vi "principal.vi"() -> ()   [LabVIEW 2018]
uses:
  <vilib>/Instr/_visa.llb/Select Event Type.ctl
  <vilib>/Instr/_visa.llb/VISA Configure Serial Port (Instr).vi
  variables_globales.vi
panel:
  out "Waveform Chart 3":dbl(graph)
  out "Waveform Chart 2":dbl(graph)
  out "Waveform Chart":dbl(graph)
  in  "Seleccione el puerto serial":refnum<visa-resource-name>
  in  "stop":bool
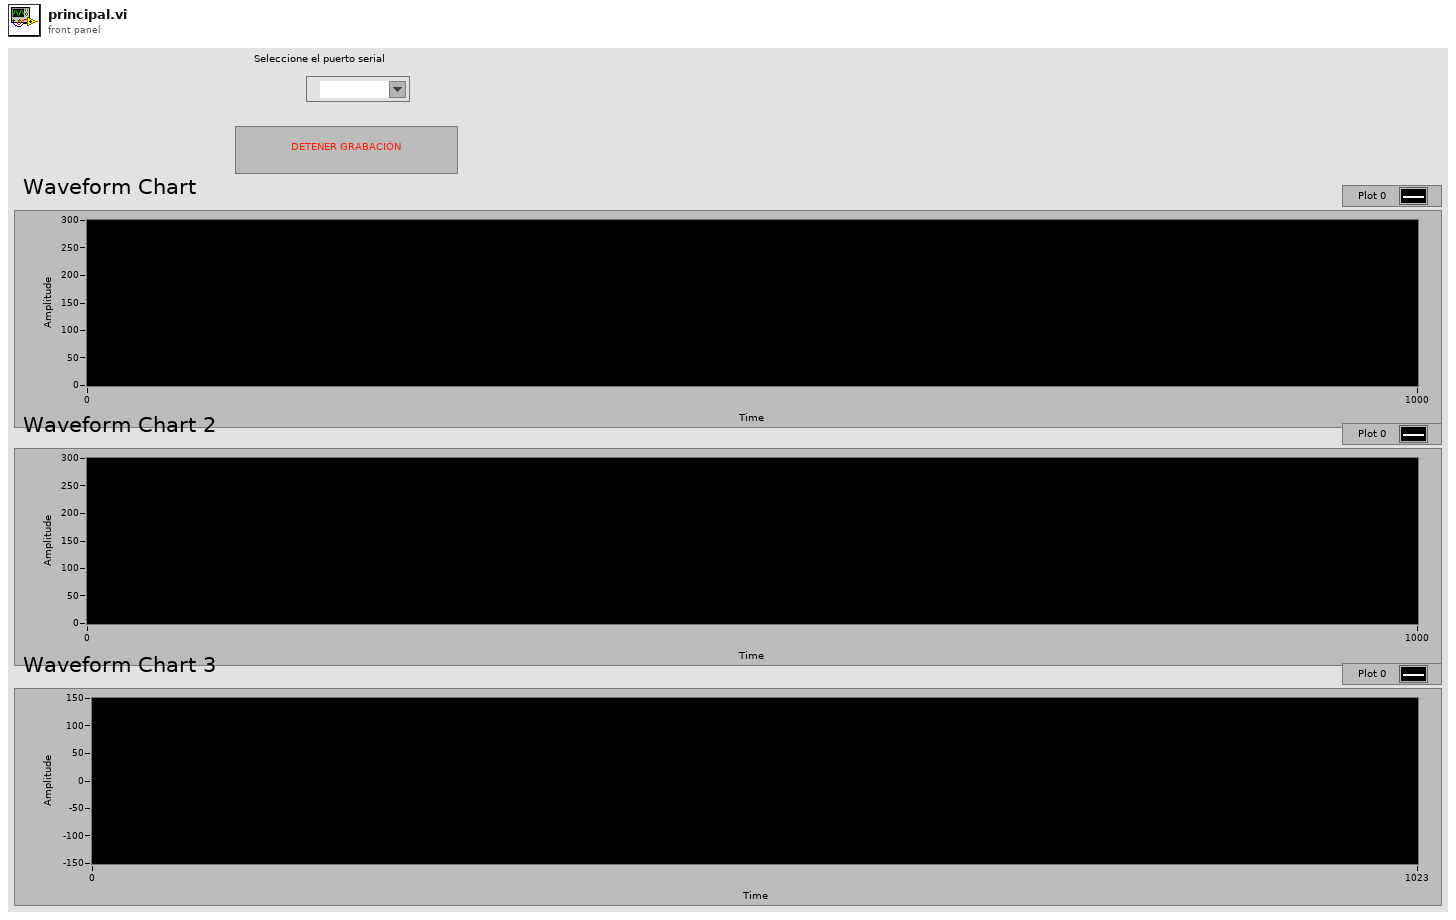
[diagram p1: front panel]
types:
  T1 = typedef "Select Event Type.ctl" = u32
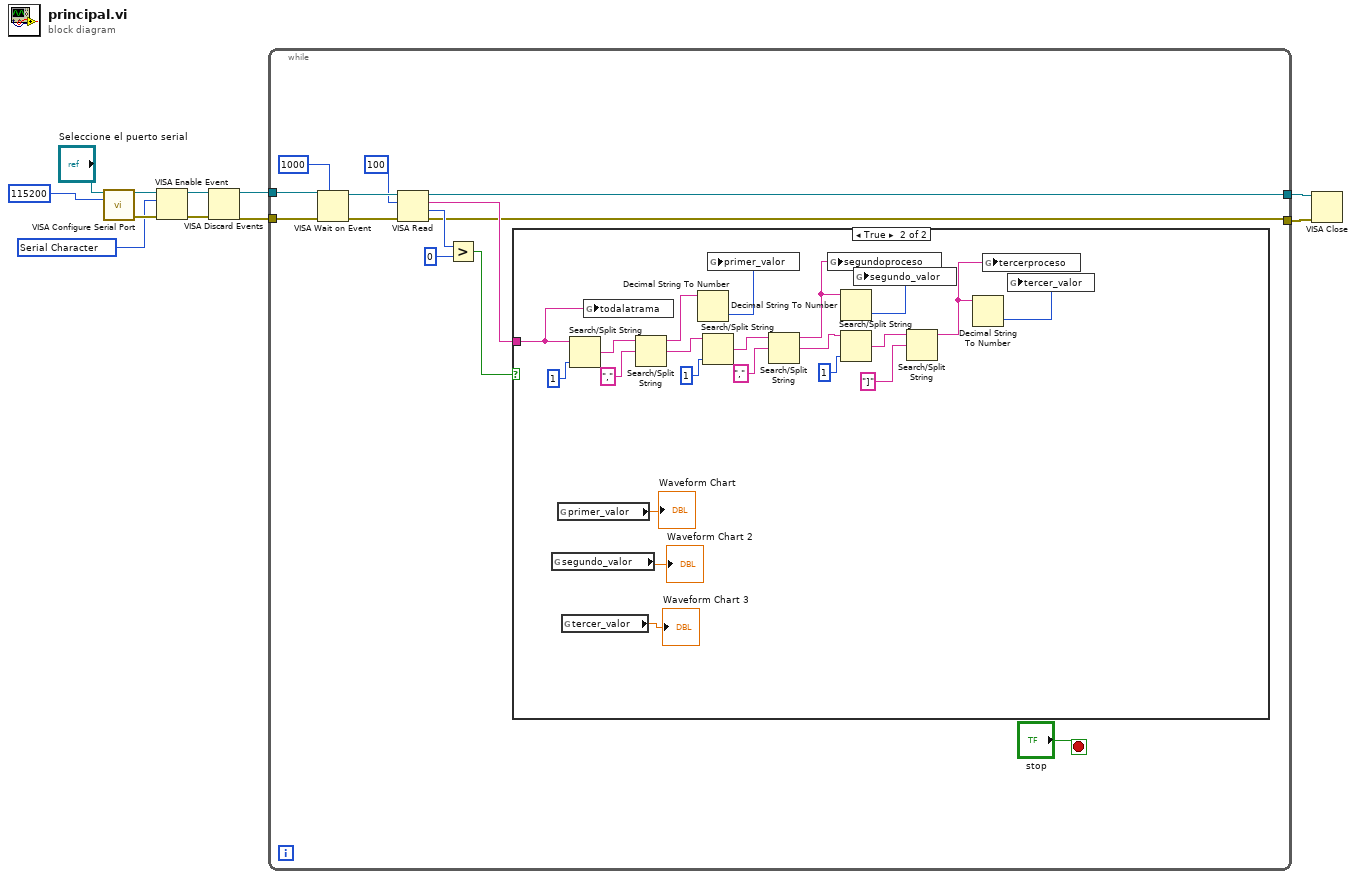
[diagram p0: block diagram]
diagram:
  w7 = T1 1073684533 items=["Service Request"=1073684491, "Trigger"=3221168138, "Clear"=1073684493, "VXI Signal"=1073684512, "VXI/VME Interrupt"=3221168161, "VXI/VME Sysfail"=1073684509, "VXI/VME Sysreset"=1073684510, "GPIB CIC"=1073684498, "GPIB Talk"=1073684499, "GPIB Listen"=1073684500, "PXI Interrupt"=1073684514, "Serial Break"=1073684515, "Serial TermChar"=1073684516, "Serial CTS"=1073684521, "Serial DSR"=1073684522, "Serial DCD"=1073684524, "Serial RI"=1073684526, "Serial Character"=1073684533, "USB Interrupt"=1073684535, "All Enabled"=1073709055] ("Event Type")
  n1 = call-poly "VISA Configure Serial Port"("VISA resource name"="Seleccione el puerto serial", "baud rate (9600)"=u32 115200) -> ("VISA resource name out"=w9:refnum<visa-resource-name>, "error out"=w8:errorcluster)  [unwired: 12 in]
  n2 = VISA Enable Event(8:w8, 10:w7, 11:w9) -> (0:w6:errorcluster, 3:w5:refnum<visa-resource-name>)  [unwired: 1 in]
  n3 = VISA Discard Events(8:w6, 11:w5) -> (0:w3:errorcluster, 3:w4:refnum<visa-resource-name>)  [unwired: 2 in]
  n4 = while {
    tunnel: w4 -> [w23]
    tunnel: w3 -> [w22]
    tunnel: [w13] -> w2
    tunnel: [w12] -> w1
    stop <- "stop" stop-if-true
    n5 = VISA Wait on Event(7:u32 1000 ("timeout (0)"), 8:w22, 11:w23) -> (0:w19:errorcluster, 3:w20:refnum<visa-resource-name>)  [unwired: 2 in, 2 out]
    n6 = VISA Read(VISA resource name=w20, byte count=u32 100, error in (no error)=w19) -> (VISA resource name out=w13:refnum<visa-resource-name>, read buffer=w14:string, return count=w17:u32, error out=w12:errorcluster)
    n7 = Greater?(x=w17, y=u32 0) -> (0:w15:bool)
    n8 = case shown="True" w15 {
      tunnel: w14 -> [_ w44]
      frame False {
      }
      frame True {
        n9 = global read "variables_globales.vi" "segundo_valor"() -> (→"Waveform Chart 2":dbl)
        n10 = global read "variables_globales.vi" "primer_valor"() -> (→"Waveform Chart":dbl)
        n11 = global read "variables_globales.vi" "tercer_valor"() -> (→"Waveform Chart 3":dbl)
        n12 = Search/Split String(string=w44, offset (0)=1) -> (match + rest of string=w43:string)  [unwired: 1 in, 2 out]
        n13 = global write "variables_globales.vi" "todalatrama"(w44) -> ()
        n14 = Search/Split String(string=w43, search string/char (-)=",") -> (substring before match=w41:string, match + rest of string=w37:string)  [unwired: 1 in, 1 out]
        n15 = Decimal String To Number(string=w41) -> (number=w32:i32)  [unwired: 2 in, 1 out]
        n16 = Search/Split String(string=w37, offset (0)=1) -> (match + rest of string=w39:string)  [unwired: 1 in, 2 out]
        n17 = global write "variables_globales.vi" "primer_valor"(w32) -> ()
        n18 = Search/Split String(string=w39, search string/char (-)=",") -> (substring before match=w28:string, match + rest of string=w33:string)  [unwired: 1 in, 1 out]
        n19 = global write "variables_globales.vi" "segundoproceso"(w28) -> ()
        n20 = Decimal String To Number(string=w28) -> (number=w27:i32)  [unwired: 2 in, 1 out]
        n21 = Search/Split String(string=w33, offset (0)=1) -> (match + rest of string=w35:string)  [unwired: 1 in, 2 out]
        n22 = global write "variables_globales.vi" "segundo_valor"(w27) -> ()
        n23 = Search/Split String(string=w35, search string/char (-)="]") -> (substring before match=w25:string)  [unwired: 1 in, 2 out]
        n24 = Decimal String To Number(string=w25) -> (number=w26:i32)  [unwired: 2 in, 1 out]
        n25 = global write "variables_globales.vi" "tercerproceso"(w25) -> ()
        n26 = global write "variables_globales.vi" "tercer_valor"(w26) -> ()
      }
    }
  }
  n27 = VISA Close(VISA resource name=w2, error in (no error)=w1) -> ()  [unwired: 1 out]
